vi "Log The Message.vi"(11 "Draw Message":refnum<class "Draw Message.lvclass">) -> (2 "log text":string="Undefined message")   [LabVIEW 2023, in "Draw Messages.lvlib" / "Draw Message.lvclass"]
uses:
  Draw Message.lvclass
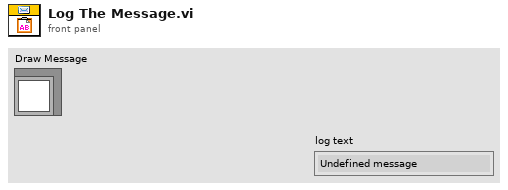
[diagram p1: front panel]
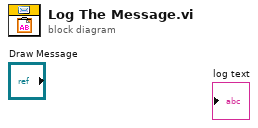
[diagram p0: block diagram]
diagram:
